vi "User events received by multiple event structures.vi"   [LabVIEW 2013]
doc: "This VI demonstrates that a user event is always received by all listeners that have subscribed to the event.\n\nRunning this VI a few times will show that the order in which the subscribers receive and respond to the event is arbitrary, so take care if you require a specific order of execution when responding to user events.\n\nThe user event can be saved into a functional global variable (FGV) so that it can be registered for events and used anywhere in your application."
panel:
  # "Demonstration that user events are received by all listeners.\n\nDr. Chris Empson\nSchool of Chemistry\nUniversity of Leeds\nUK\n\nc.j.empson@leeds.ac.uk\nTwitter: @monty_mcmont\n\n(CTRL+E to see block diagram!)"
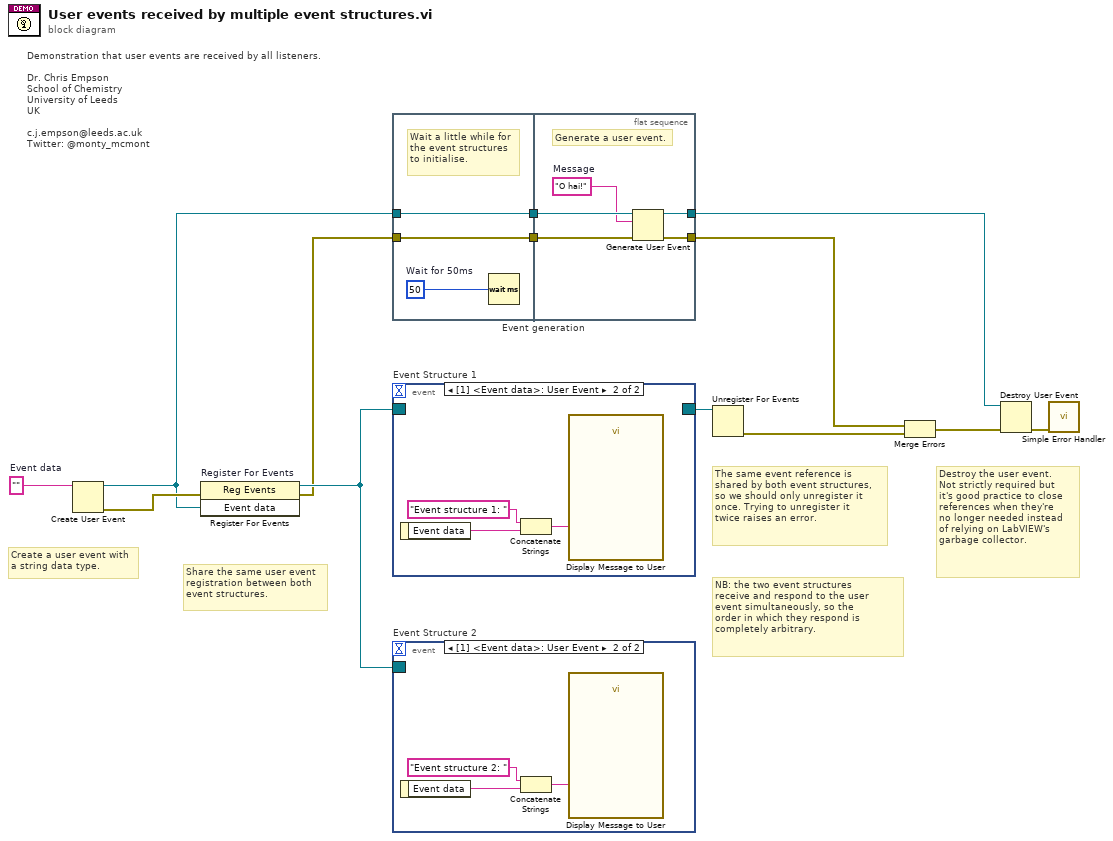
[diagram p0: block diagram]
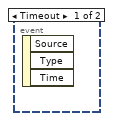
[diagram p2: hidden frame]
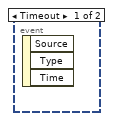
[diagram p3: hidden frame]
diagram:
  w4 = ""  # Event data
  # "NB: the two event structures \nreceive and respond to the user\nevent simultaneously, so the \norder in which they respond is\ncompletely arbitrary."
  # "Create a user event with\na string data type."
  # "Destroy the user event.\nNot strictly required but\nit's good practice to close\nreferences when they're\nno longer needed instead\nof relying on LabVIEW's\ngarbage collector."
  # "Share the same user event \nregistration between both\nevent structures."
  # "The same event reference is\nshared by both event structures,\nso we should only unregister it\nonce. Trying to unregister it\ntwice raises an error."
  # "Demonstration that user events are received by all listeners.\n\nDr. Chris Empson\nSchool of Chemistry\nUniversity of Leeds\nUK\n\nc.j.empson@leeds.ac.uk\nTwitter: @monty_mcmont"
  n1 = Create User Event(user event datatype=w4) -> (user event=w12:refnum<user-event>, error out=w13:errorcluster)  [unwired: 1 in]
  n2 = register-events "Register For Events"(error in=w13, w12) -> (reference out=w3:refnum<event-registration>, error out=w1:errorcluster)  [unwired: 1 in]
  n3 = flat-sequence "Event generation" {
    tunnel: w12 -> [w15]
    tunnel: [w15] -> w11
    tunnel: [w14] -> w2
    tunnel: w1 -> [w14]
    tunnel: w11 -> [w21]
    tunnel: [w20] -> w8
    tunnel: [w19] -> w6
    tunnel: w2 -> [w17]
    frame #0 {
      w16 = u32 50  # Wait for 50ms
      # "Wait a little while for\nthe event structures\nto initialise."
      n4 = Wait (ms)(milliseconds to wait=w16) -> ()  [unwired: 1 out]
    }
    frame #1 {
      w18 = "O hai!"  # Message
      # "Generate a user event."
      n5 = Generate User Event(user event=w21, event data cluster=w18, error in=w17) -> (user event out=w19:refnum<user-event>, error out=w20:errorcluster)  [unwired: 1 in]
    }
  }
  n6 = event "Event Structure 1" shown="[1] <Event data>: User Event" {
    selector: w3 -> [_ _]
    dyn-events: [_ _] -> w10
    timeout: _ -> [_ _]
    event Timeout {
      n7 = event-data() -> ()  [unwired: 1 in, 3 out]
    }
    event User Event {
      n8 = event-data() -> ("Event data"=w23:string)  [unwired: 1 in]
      n9 = Concatenate Strings("Event structure 1: " ("Message"), w23) -> (w22:string)
      n10 = call "Display Message to User"("Message"=w22) -> ()  [unwired: 9 in, 2 out]
    }
  }
  n11 = event "Event Structure 2" shown="[1] <Event data>: User Event" {
    selector: w3 -> [_ _]
    dyn-events: _ -> [_ _]
    timeout: _ -> [_ _]
    event Timeout {
      n12 = event-data() -> ()  [unwired: 1 in, 3 out]
    }
    event User Event {
      n13 = event-data() -> ("Event data"=w26:string)  [unwired: 1 in]
      n14 = Concatenate Strings("Event structure 2: " ("Message"), w26) -> (w25:string)
      n15 = call "Display Message to User"("Message"=w25) -> ()  [unwired: 9 in, 2 out]
    }
  }
  n16 = Unregister For Events(event registration refnum=w10) -> (error out=w9:errorcluster)  [unwired: 1 in]
  n17 = Merge Errors "Merge Errors"(w8, w9) -> (w7:errorcluster)
  n18 = Destroy User Event(user event=w6, error in=w7) -> (error out=w5:errorcluster)
  n19 = call <vilib>:"Simple Error Handler.vi"("error in (no error)"=w5) -> ()  [unwired: 4 in, 5 out]
